vi "Logging Cases.vi"(0 "Logging queue":refnum<queue>, 1 "Channel info":T1, 3 "Number of files closed in":u32, 5 "Logging queue element in":T6={"Imaging Protocol"=enum."Live Imaging", "Number of Trials"=0, "Frame Size"=512, "# Averaged frames"=0, "Dwell time (us)"=0.0, "Index of Z-plane"=0, "Timelapse?"=FALSE, "Logging process is active"=FALSE, "Speed logging enabled"=FALSE, "tdms file ref"=refnum, "path"=path "", "Trial Number"=0, "Expected # points acquired"=FALSE, "Manually stopped"=FALSE, "Ch0 data"=[], "Ch1 data"=[], "Last trial"=FALSE, "Points acquired"={"Ch0 last trial"=0, "Ch1 last trial"=0, "All trials"=0}} {"Frame Size" items=["100X100"=100, "128X128"=128, "200X200"=200, "256X256"=256, "512X512"=512, "1024x1024"=1024, "2048x2048"=2048]; "Dwell time (us)" format="%#.6g"}, 7 "UI queue":refnum<queue>, 9 "Data-gen queue":T5, 11 "error in":errorcluster, 12 "Live graph data queue in":T2, 14 "Image array":T3) -> (6 "Number of TDMS files closed":u32, 15 "error out":errorcluster)   [LabVIEW 2013]
uses:
  Typedefs/Logging queue element.ctl
  Typedefs/Imaging Protocols enum.ctl
  Typedefs/Frame Size.ctl
  Typedefs/Acquired points count.ctl
  Typedefs/ROI File Generator Queue Ref.ctl
  User Interface/Queue/Live graphs queue/Typedefs/Live imaging queue element.ctl
  <vilib>/vision/Image Controls.llb/IMAQ Image.ctl
  User Interface/Typedefs/Live graph data queue ref.ctl
  User Interface/Queue/Message Queue/Typedefs/Message Cluster.ctl
panel:
  out "Number of points in completed standard frame":i32
  out "Peak # points received":dbl
  out "# points received":i32
  # "<-- For debugging only"
  # "<-- For debugging only"
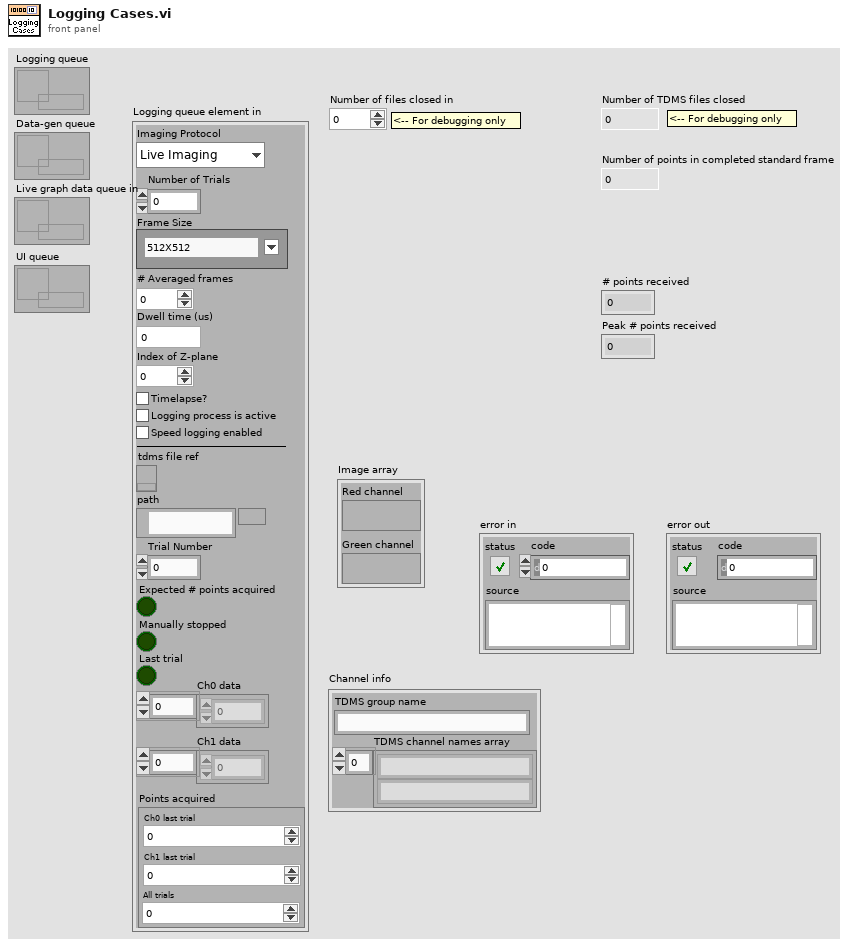
[diagram p1: front panel]
types:
  T1 = cluster{"TDMS group name":string, "TDMS channel names array":string[]}
  T2 = typedef "Live graph data queue ref.ctl" = refnum<queue>
  T3 = typedef "Live imaging queue element.ctl" = cluster{"Red channel":T4, "Green channel":T4}
  T4 = typedef "IMAQ Image.ctl" = refnum<image>
  T5 = typedef "ROI File Generator Queue Ref.ctl" = refnum<queue>
  T6 = typedef "Logging queue element.ctl" = cluster{"Imaging Protocol":T7, "Number of Trials":u16, "Frame Size":T8, "# Averaged frames":u16, "Dwell time (us)":dbl, "Index of Z-plane":i32, "Timelapse?":bool, "Logging process is active":bool, "Speed logging enabled":bool, "tdms file ref":refnum<k34>, "path":path, "Trial Number":i32, "Expected # points acquired":bool, "Manually stopped":bool, "Ch0 data":u32[], "Ch1 data":u32[], "Last trial":bool, "Points acquired":T9}
  T7 = typedef "Imaging Protocols enum.ctl" = enum16{"AOL Z-Stack", "Motor Z Stack", "Functional Acquisition", "Single Plane Acquisition", "Volume Acquisition", "Live Imaging", "Live Plane Imaging", "Live Volume Imaging"}
  T8 = typedef "Frame Size.ctl" = u16
  T9 = typedef "Acquired points count.ctl" = cluster{"Ch0 last trial":u64, "Ch1 last trial":u64, "All trials":u64}
  T10 = typedef "Frame data dual cluster.ctl" = cluster{"Red channel frame":dbl[], "Green channel frame":dbl[]}
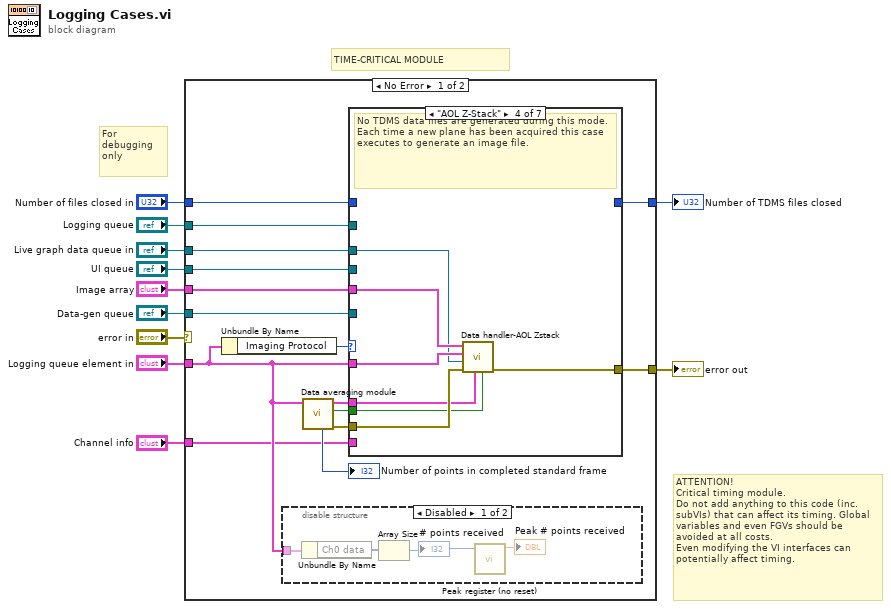
[diagram p0: block diagram]
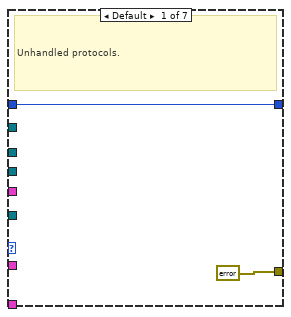
[diagram p2: hidden frame]
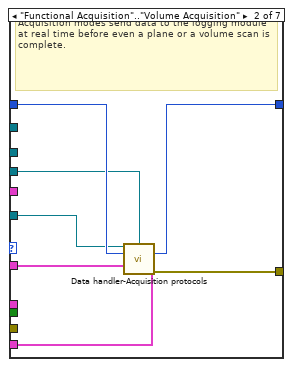
[diagram p3: hidden frame]
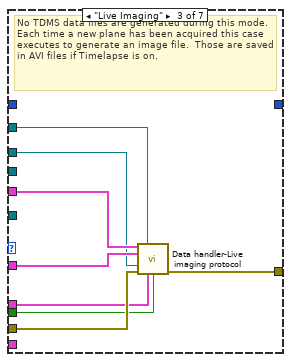
[diagram p4: hidden frame]
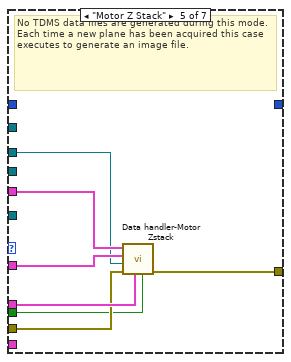
[diagram p5: hidden frame]
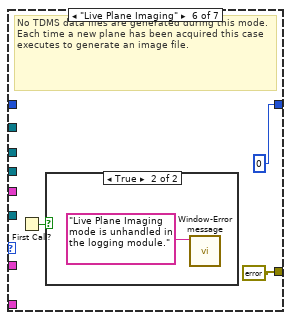
[diagram p6: hidden frame]
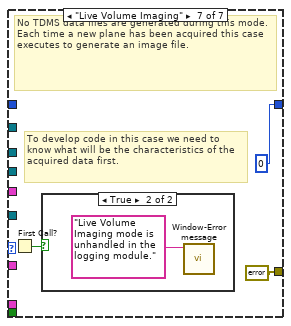
[diagram p8: hidden frame]
diagram:
  # "TIME-CRITICAL MODULE"
  # "ATTENTION!\nCritical timing module.\nDo not add anything to this code (inc. subVIs) that can affect its timing. Global variables and even FGVs should be avoided at all costs.\nEven modifying the VI interfaces can potentially affect timing."
  # "For debugging only"
  n1 = case shown="No Error" "error in" {
    selector: "error in" -> [_ w70]
    tunnel: "Number of files closed in" -> [w26 _]
    tunnel: [w25 _] -> w10
    tunnel: "Data-gen queue" -> [w24 _]
    tunnel: [w23 w70] -> w8
    tunnel: "Logging queue element in" -> [w16 _]
    tunnel: "Image array" -> [w21 _]
    tunnel: "Live graph data queue in" -> [w20 _]
    tunnel: "Channel info" -> [w14 _]
    tunnel: "Logging queue" -> [w13 _]
    tunnel: "UI queue" -> [w12 _]
    frame No Error {
      n2 = Unbundle By Name(w16) -> ("Imaging Protocol"=w22:T7)
      n3 = disable-structure shown="Disabled" {
        disable-tunnel: w16 -> [w66 _]
        frame Disabled {
          n4 = Unbundle By Name(w66) -> ("Ch0 data"=w67:u32[])
          n5 = Array Size(array=w67) -> (size(s)=w68:i32)
          "# points received" <- w68
          n6 = call "Peak register (no reset).vi"("Value in"=w68) -> ("Registered peak value"=→"Peak # points received":dbl)  [unwired: 10 in]
        }
        frame Enabled {
        }
      }
      n7 = call "Data averaging module.vi"("Logging queue element in"=w16) -> ("error out"=w19:errorcluster, "Standard Frame completed/generate image"=w17:bool, "Single Frame Data"=w18:T10, "Number of points in completed standard frame"=→"Number of points in completed standard frame":i32)  [unwired: 7 in]
      n8 = case shown="\"AOL Z-Stack\"" w22 {
        tunnel: w26 -> [w28 w35 _ _ _ _ _]
        tunnel: [w28 w31 _ _ _ u32 0 ("Number of files closed in") u32 0 ("Number of files closed in")] -> w25
        tunnel: w24 -> [_ w34 _ _ _ _ _]
        tunnel: [errorcluster {"status"=FALSE, "code"=0, "source"=""} ("error out") w33 w41 w48 w56 errorcluster {"status"=FALSE, "code"=0, "source"=""} ("error out") errorcluster {"status"=FALSE, "code"=0, "source"=""} ("error out")] -> w23
        tunnel: w16 -> [_ w32 w42 w49 w55 _ _]
        tunnel: w21 -> [_ _ w43 w50 w57 _ _]
        tunnel: w20 -> [_ _ w40 w44 w51 _ _]
        tunnel: w19 -> [_ _ w39 w47 w53 _ _]
        tunnel: w18 -> [_ _ w38 w46 w54 _ _]
        tunnel: w17 -> [_ _ w37 w45 w52 _ _]
        tunnel: w14 -> [_ w30 _ _ _ _ _]
        tunnel: w13 -> [_ _ w36 _ _ _ _]
        tunnel: w12 -> [_ w29 _ _ _ _ _]
        frame Default {
          # "Unhandled protocols."
        }
        frame "Functional Acquisition".."Volume Acquisition" {
          # "Acquisition modes send data to the logging module at real time before even a plane or a volume scan is complete."
          n9 = call "Data handler-Acquisition protocols.vi"("Data-gen queue"=w34, "UI queue"=w29, "Channel info"=w30, "Number of files closed in in"=w35, "Logging queue element in"=w32) -> ("Number of files closed out"=w31:u32, "error out"=w33:errorcluster)  [unwired: 9 in]
        }
        frame "Live Imaging" {
          # "No TDMS data files are generated during this mode.  Each time a new plane has been acquired this case executes to generate an image file.  Those are saved in AVI files if Timelapse is on."
          n10 = call "Data handler-Live imaging protocol.vi"("Image array"=w43, "Logging queue"=w36, "Logging queue element in"=w42, "Live graph data queue in"=w40, "error in (no error)"=w39, "Single Frame Data"=w38, "Frame completed/generate image"=w37) -> ("error out"=w41:errorcluster)  [unwired: 8 in]
        }
        frame "AOL Z-Stack" {
          # "No TDMS data files are generated during this mode. Each time a new plane has been acquired this case executes to generate an image file."
          n11 = call "Data handler-AOL Zstack.vi"("Save image"=w45, "Single Frame Data"=w46, "error in (no error)"=w47, "Live graph data queue in"=w44, "Logging queue element in"=w49, "Image array"=w50) -> ("error out"=w48:errorcluster)  [unwired: 5 in]
        }
        frame "Motor Z Stack" {
          # "No TDMS data files are generated during this mode. Each time a new plane has been acquired this case executes to generate an image file."
          n12 = call "Data handler-Motor Zstack.vi"("Save image"=w52, "Single Frame Data"=w54, "error in (no error)"=w53, "Live graph data queue in"=w51, "Logging queue element in"=w55, "Image array"=w57) -> ("error out"=w56:errorcluster)  [unwired: 5 in]
        }
        frame "Live Plane Imaging" {
          # "No TDMS data files are generated during this mode. Each time a new plane has been acquired this case executes to generate an image file."
          n13 = First Call?() -> (First Call?: T/F=w58:bool)
          n14 = case shown="True" w58 {
            frame False {
            }
            frame True {
              n15 = call "Window-Error message.vi"("Message"="Live Plane Imaging mode is unhandled in the logging module." ("message")) -> ()  [unwired: 10 in, 1 out]
            }
          }
        }
        frame "Live Volume Imaging" {
          # "To develop code in this case we need to know what will be the characteristics of the acquired data first."
          # "No TDMS data files are generated during this mode. Each time a new plane has been acquired this case executes to generate an image file."
          n16 = First Call?() -> (First Call?: T/F=w62:bool)
          n17 = case shown="True" w62 {
            frame False {
            }
            frame True {
              n18 = call "Window-Error message.vi"("Message"="Live Volume Imaging mode is unhandled in the logging module." ("message")) -> ()  [unwired: 10 in, 1 out]
            }
          }
        }
      }
    }
    frame Error {
    }
  }
  "Number of TDMS files closed" <- w10
  "error out" <- w8
